vi "Get AF Control Parameter.vi"(8 "error in (no error)":errorcluster {"code" format="%.0x"}, 9 "Parameter Number (1)":i32=1, 10 "Device Number (1)":i32=1, 11 "VISA Resource Name":refnum<visa-resource-name>) -> (0 "error out":errorcluster {"code" format="%.0x"}, 2 "Data":i32=1, 3 "VISA Resource Name Out":refnum<visa-resource-name>)   [LabVIEW 2020, in "Olympus IX BX Series.lvlib"]
doc: "Gets the AF control parameter."
uses:
  Olympus IX BX Series.lvlib
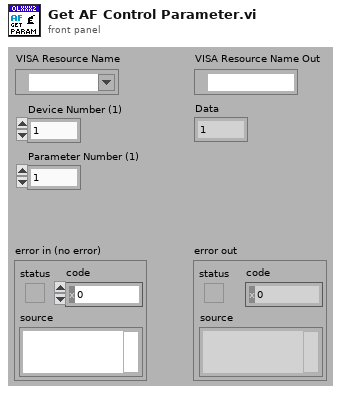
[diagram p1: front panel]
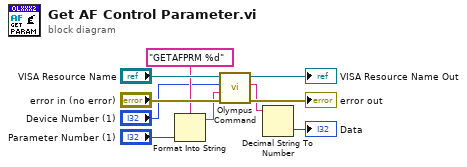
[diagram p0: block diagram]
diagram:
  n1 = Format Into String(format string="GETAFPRM %d", "Parameter Number (1)") -> (resulting string=w8:string)  [unwired: 2 in, 1 out]
  n2 = call "Olympus Command.vi"("error in (no error)"="error in (no error)", "Command string"=w8, "Device Number (1)"="Device Number (1)", "VISA Resource Name"="VISA Resource Name") -> ("error out"=→"error out":errorcluster, "Result"=w2:string, "VISA Resource Name Out"=→"VISA Resource Name Out":refnum<visa-resource-name>)  [unwired: 5 in]
  n3 = Decimal String To Number(string=w2) -> (number=→"Data":i32)  [unwired: 2 in, 1 out]
